vi "Slice Engine.vi"(7 "Table Stages":T3={"X Stage"={"Position"=0.0, "Is.Enabled?"=FALSE, "Is.Connected?"=FALSE, "Device SN"="45876425", "AccelerationMaximum"=20.0, "VelocityMaximum"=20.0, "Acceleration"=15.0, "Velocity"=18.0, "waitTimeout (ms)"=500000, "Model"=enum."None", "Is.Homed?"=FALSE, "MOVE"=FALSE}, "Y Stage"={"Position"=0.0, "Is.Enabled?"=FALSE, "Is.Connected?"=FALSE, "Device SN"="45995820", "AccelerationMaximum"=20.0, "VelocityMaximum"=20.0, "Acceleration"=15.0, "Velocity"=18.0, "waitTimeout (ms)"=5000000, "Model"=enum."None", "Is.Homed?"=FALSE, "MOVE"=FALSE}, "Z Stage"={"Position"=0.0, "Is.Enabled?"=FALSE, "Is.Connected?"=FALSE, "Device SN"="49103464", "AccelerationMaximum"=0.0, "VelocityMaximum"=0.0, "Acceleration"=0.0, "Velocity"=0.0, "waitTimeout (ms)"=0, "Model"=enum."None", "Is.Homed?"=FALSE, "MOVE"=FALSE}, "Attenuator"={"Position"=0.0, "Is.Enabled?"=FALSE, "Is.Connected?"=FALSE, "Device SN"="45876539", "AccelerationMaximum"=0.0, "VelocityMaximum"=0.0, "Acceleration"=0.0, "Velocity"=0.0, "waitTimeout (ms)"=0, "Model"=enum."None", "Is.Homed?"=FALSE, "MOVE"=FALSE}}, 8 "error in (no error)":errorcluster, 9 "Vibratome":T1={"Pre Cut Dwell [s]"=0.0, "Blade Frequency [RPM]"=0, "Slice Speed [mm/s]"=0.0, "Post Cut Dwell [s]"=0.0, "Ramp Time [s]"=0.0, "Start X [mm]"=0.0, "Start Y [mm]"=0.0, "Slice Length [mm]"=0.0, "Slice Axis"=enum."X Axis", "Controller VISA Ref"="COM4", "Blade Frequency [Hz]"=0, "Analog Out Channel"="GalvoCtrl/ao0,GalvoCtrl/ao1", "Pixel Clock Source"="/GalvoCtrl/PFI0", "Vib version"=enum."Vibratome1"}, 10 "Action":string="Init", 11 "Last Slice?":bool) -> (0 "error out":errorcluster)   [LabVIEW 2018]
uses:
  Controls/Translation Stage Parameters.ctl
  Hardware Mfg/Thorlabs Translation Stages/Controls/Translation Stage Cluster.ctl
  Controls/Translation Stage Types.ctl
  Controls/Vibratome Parameters.ctl
  type defines/vibratome.ctl
  Controls/Queue Manager Actions.ctl
  Controls/QueueNames.ctl
  Controls/Set Get Controls.ctl
  Hardware Mfg/Thorlabs Translation Stages/Controls/Motion Translation Module Control2.ctl
  Controls/FGV Actions.ctl
  Hardware Mfg/Thorlabs Translation Stages/Controls/Motion Translation Module Control.ctl
  Controls/vibratome3 control.ctl
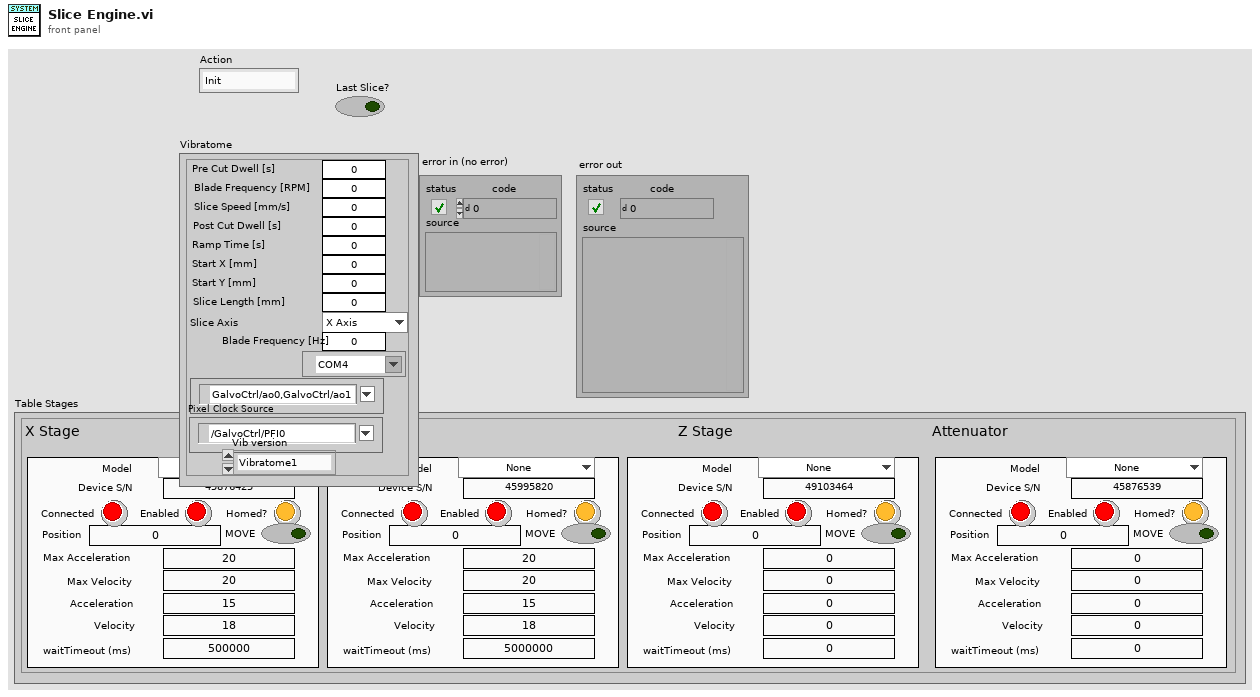
[diagram p1: front panel]
types:
  T1 = typedef "Vibratome Parameters.ctl" = cluster{"Pre Cut Dwell [s]":dbl, "Blade Frequency [RPM]":u16, "Slice Speed [mm/s]":dbl, "Post Cut Dwell [s]":dbl, "Ramp Time [s]":dbl, "Start X [mm]":dbl, "Start Y [mm]":dbl, "Slice Length [mm]":dbl, "Slice Axis":enum16{"X Axis", "Y Axis", "Z Axis"}, "Controller VISA Ref":refnum<visa-resource-name>, "Blade Frequency [Hz]":u16, "Analog Out Channel":tag, "Pixel Clock Source":tag, "Vib version":T2}
  T2 = typedef "vibratome.ctl" = enum16{"Vibratome1", "Vibratome3"}
  T3 = typedef "Translation Stage Parameters.ctl" = cluster{"X Stage":T4, "Y Stage":T4, "Z Stage":T4, "Attenuator":T4}
  T4 = typedef "Translation Stage Cluster.ctl" = cluster{"Position":dbl, "Is.Enabled?":bool, "Is.Connected?":bool, "Device SN":string, "AccelerationMaximum":dbl, "VelocityMaximum":dbl, "Acceleration":dbl, "Velocity":dbl, "waitTimeout (ms)":i32, "Model":T5, "Is.Homed?":bool, "MOVE":bool}
  T5 = typedef "Translation Stage Types.ctl" = enum16{"None", "Thorlabs LTS", "Thorlabs MLJ"}
  T6 = typedef "QueueNames.ctl" = enum16{"Main GUI", "Main Scan Processor", "Main Processing", "Main Saving", "Main Display", "Main Table Stage GUI", "Main Table Stage Proc.", "Scan Engine", "Vibratome GUI", "Vibratome Processor", "Slice Engine"}
  T7 = typedef "Queue Manager Actions.ctl" = enum16{"Init", "Enqueue", "Enqueue All", "Preview Queue", "Dequeue", "Get Status", "Flush Queue", "Flush All Queues", "Release All Queues", "Release Queue", "Enqueue at Opposite End"}
  T8 = typedef "Set Get Controls.ctl" = enum16{"Set", "Get"}
  T9 = typedef "Motion Translation Module Control.ctl" = enum16{"Init", "Home", "Status", "Velocity/Accel", "Position", "Jog", "Stop", "Uninit", "Enable", "Disable"}
  T10 = typedef "Motion Translation Module Control2.ctl" = enum16{"Init", "Home", "Status", "Velocity/Accel", "Position", "Jog", "Stop", "Uninit", "Enable", "Disable"}
  T11 = typedef "FGV Actions.ctl" = enum16{"Init", "Set", "Get", "Clear"}
  T12 = enum16{"Set Configuration", "Get Configuration", "Enable Motor", "Disable Motor", "Get Status", "Open Session", "Close Session", "Set Limits", "Get Limits"}
  T13 = cluster{"Source for Velocity":enum16{"Interface", "Voltage (AI)", "PWM (AI)", "Current Target (AI)", "Current Target w/ Preset (AI)"}, "Mode":enum16{"Continuous", "Stepper Motor", "Analog Position Ctrl", "Encoder"}, "Target Velocity [RPM]":i16}
  T14 = typedef "vibratome3 control.ctl" = enum16{"Init", "Configure channel", "Write waveform", "Start", "Stop", "Finish?", "Uninit"}
  T15 = typedef "Motion Translation Module Control.ctl" = enum16{"Uninit", "Measure power", "Move angle", "Gen angles", "Init cage", "Init PM"}
  T16 = typedef "MessagePacket.ctl" = cluster{"Message":string, "Parameter":variant}
  T17 = typedef "Translation Stage Quick Status.ctl" = cluster{"Is.Enabled?":bool, "Is.Connected?":bool, "Is.Homed?":bool}
  T18 = typedef "ScanType.ctl" = enum16{"Single Frame", "Continuous Frame", "ROI Line", "Vibratome", "Mosaic", "Mosaic + Slice"}
  T19 = enum16{"Left Button", "Center Button", "Right Button", "Window Close"}
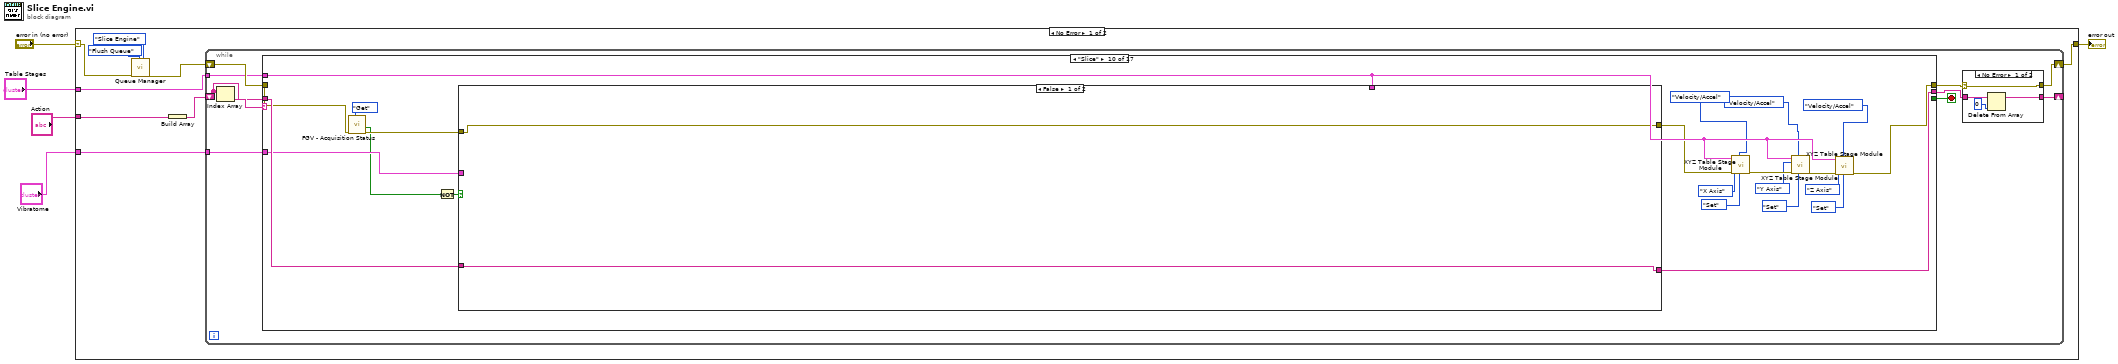
[diagram p0: block diagram]
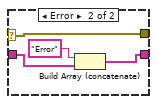
[diagram p2: hidden frame]
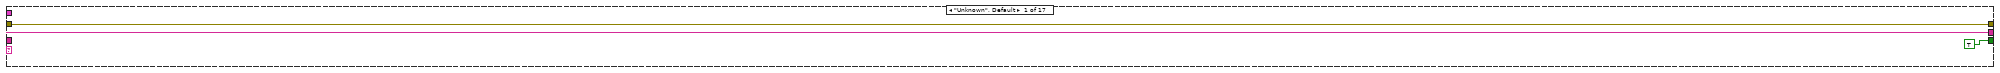
[diagram p3: hidden frame]
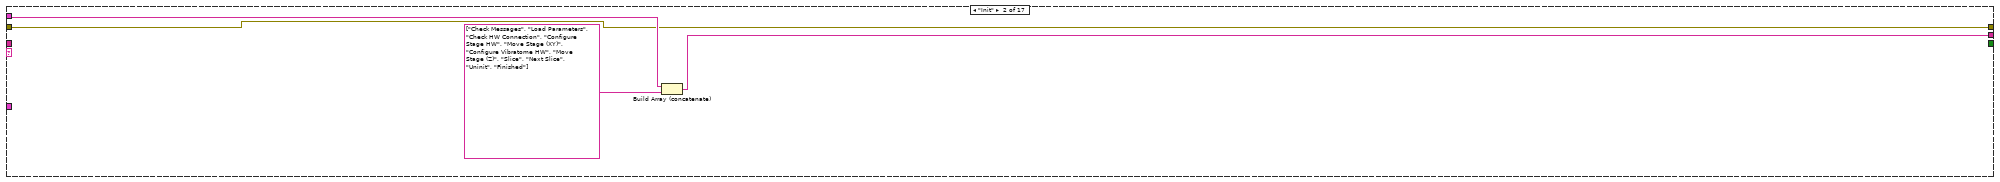
[diagram p4: hidden frame]
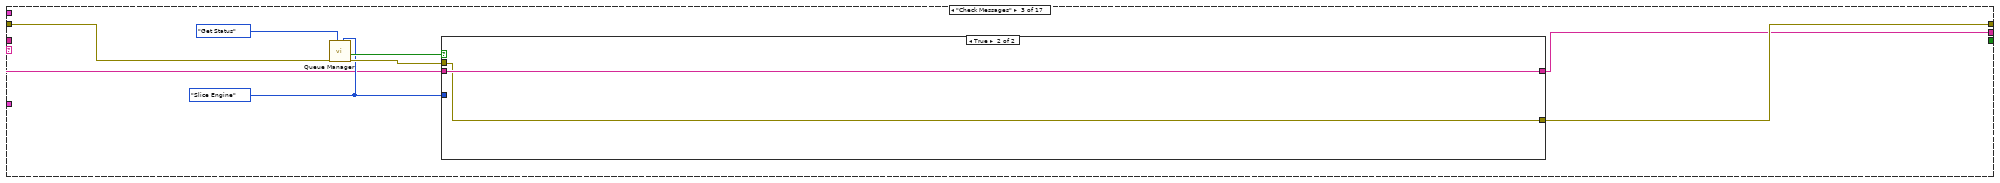
[diagram p5: hidden frame]
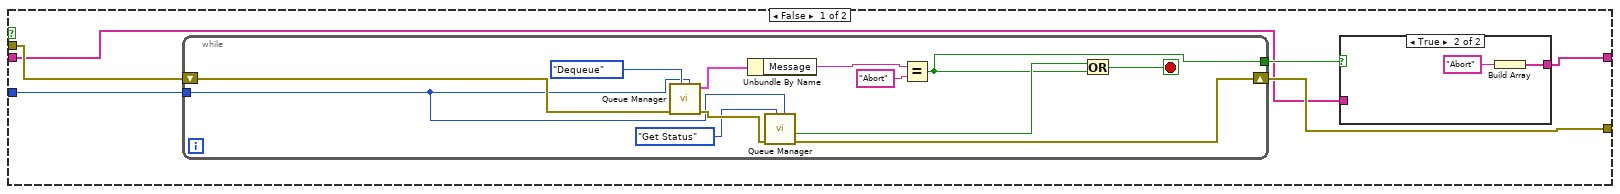
[diagram p6: hidden frame]
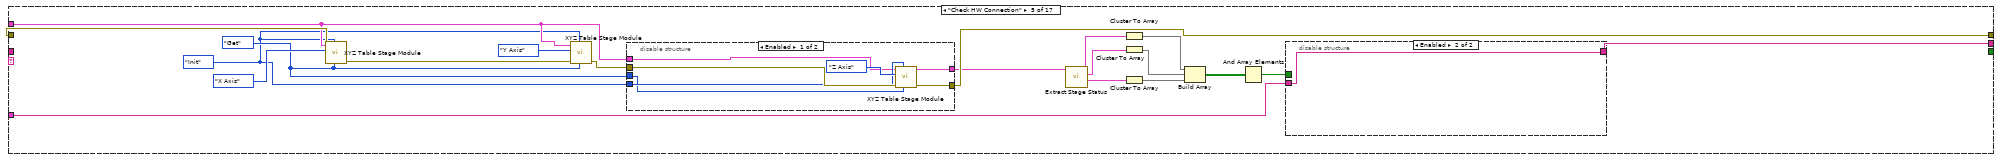
[diagram p9: hidden frame]
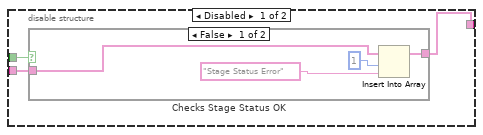
[diagram p10: hidden frame]
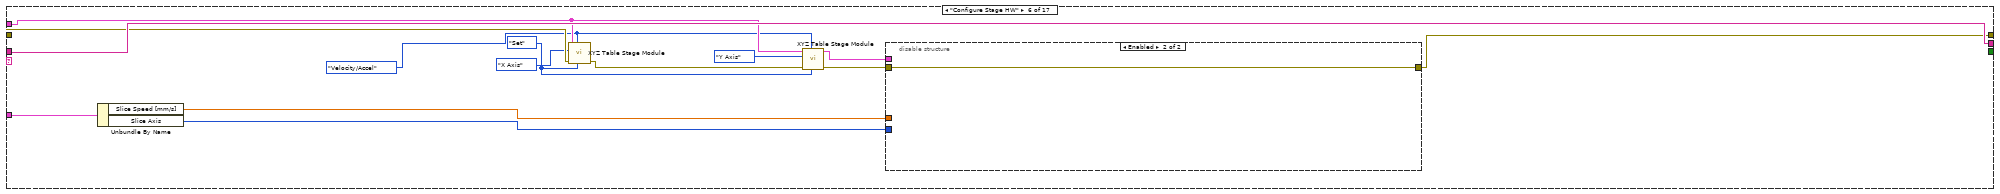
[diagram p13: hidden frame]
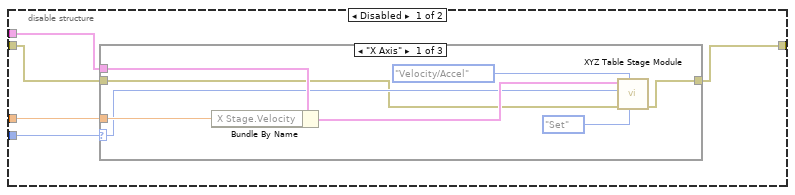
[diagram p14: hidden frame]
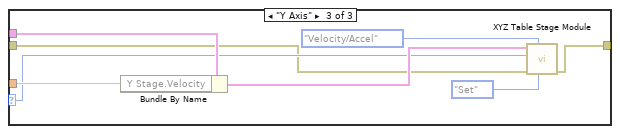
[diagram p16: hidden frame]
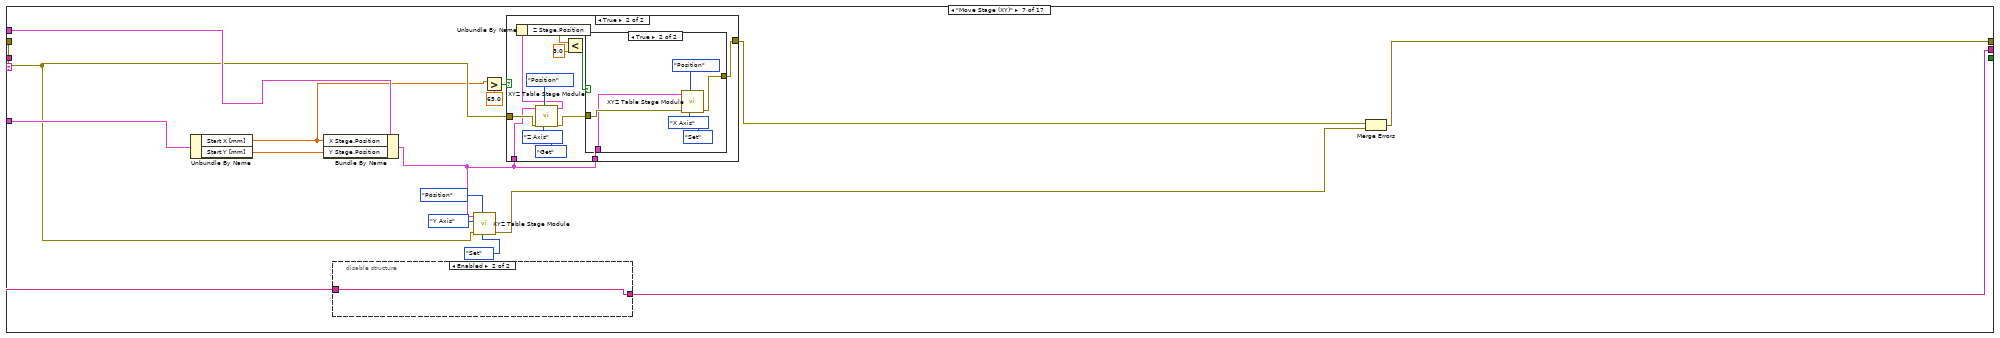
[diagram p17: hidden frame]
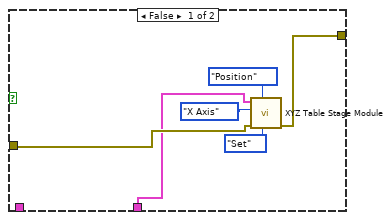
[diagram p18: hidden frame]
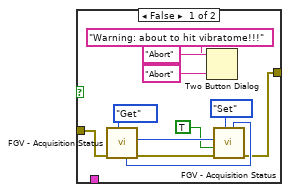
[diagram p19: hidden frame]
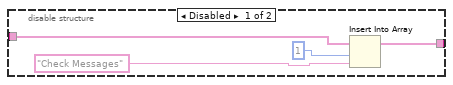
[diagram p20: hidden frame]
diagram:
  n1 = case shown="No Error" "error in (no error)" {
    selector: "error in (no error)" -> [w10 w540]
    tunnel: [w11 w540] -> w4
    tunnel: "Action" -> [w9 _]
    tunnel: "Table Stages" -> [w7 _]
    tunnel: "Vibratome" -> [w6 _]
    frame No Error {
      n2 = call "Queue Manager.vi"("Queue Name"=QueueNames."Slice Engine", "Action"=Queue_Manager_Actions."Flush Queue", "Error In"=w10) -> ("Error Out"=w8:errorcluster)  [unwired: 4 in, 4 out]
      n3 = Build Array(w9) -> (w12:string[])
      n4 = while {
        shift-right: [w19] -> _
        shift-left: w12 -> [w18]
        shift-right: [w21] -> w11
        shift-left: w8 -> [w24]
        tunnel: w7 -> [w17]
        tunnel: w6 -> [w16]
        stop <- w15 stop-if-true
        n5 = Index Array(array=w18) -> (element=w23:string)  [unwired: 1 in]
        n6 = case shown="\"Slice\"" w23 {
          tunnel: w24 -> [w34 w36 w47 w71 w92 w123 w151 w210 w214 w238 w333 w376 w394 w418 w422 w451 w538]
          tunnel: w18 -> [w35 w39 w41 w72 w76 w124 w163 w211 w213 w241 w336 w379 w391 w415 w420 w452 w539]
          tunnel: [w35 w38 w40 w72 w77 w124 w162 w211 w212 w240 w335 w378 w391 w416 w419 w452 w539] -> w20
          tunnel: [w34 w36 w42 w71 w91 w114 w161 w204 w214 w239 w334 w376 w392 w418 w423 w450 w537] -> w22
          tunnel: w17 -> [_ _ _ _ w74 w113 w160 _ _ w236 w331 _ w390 _ _ w449 _]
          tunnel: w16 -> [_ _ _ _ _ w112 w159 w206 _ w237 w332 _ w389 _ _ _ _]
          tunnel: [TRUE _ _ _ _ _ _ _ _ _ _ _ _ _ _ _ TRUE] -> w15
          frame "Unknown", Default {
          }
          frame "Init" {
            n7 = Build Array (concatenate)(w39, string[] ["Check Messages", "Load Parameters", "Check HW Connection", "Configure Stage HW", "Move Stage (XY)", "Configure Vibratome HW", "Move Stage (Z)", "Slice", "Next Slice", "Uninit", "Finished"]) -> (w38:string[])
          }
          frame "Check Messages" {
            w43 = QueueNames."Slice Engine" ("Queue Name")
            n8 = call "Queue Manager.vi"("Queue Name"=w43, "Action"=Queue_Manager_Actions."Get Status", "Error In"=w47) -> ("Error Out"=w44:errorcluster, "Empty?"=w45:bool)  [unwired: 4 in, 3 out]
            n9 = case shown="True" w45 {
              tunnel: w44 -> [w53 w69]
              tunnel: w43 -> [w52 _]
              tunnel: [w51 w69] -> w42
              tunnel: w41 -> [w49 w70]
              tunnel: [w48 w70] -> w40
              frame False {
                n10 = while {
                  tunnel: w52 -> [w64]
                  shift-right: [w65] -> w51
                  shift-left: w53 -> [w68]
                  tunnel: [w57] -> w50
                  stop <- w58 stop-if-true
                  n11 = call "Queue Manager.vi"("Queue Name"=w64, "Action"=Queue_Manager_Actions."Dequeue", "Error In"=w68) -> ("Error Out"=w66:errorcluster, "Message Packet [Out]"=w62:T16)  [unwired: 4 in, 3 out]
                  n12 = Unbundle By Name(w62) -> ("Message"=w61:string)
                  n13 = call "Queue Manager.vi"("Queue Name"=w64, "Action"=Queue_Manager_Actions."Get Status", "Error In"=w66) -> ("Error Out"=w65:errorcluster, "Empty?"=w59:bool)  [unwired: 4 in, 3 out]
                  n14 = Equal?(x=w61, y="Abort") -> (x = y?=w57:bool)
                  n15 = Or(x=w59, y=w57) -> (x .or. y?=w58:bool)
                }
                n16 = case shown="True" w50 {
                  tunnel: w49 -> [w54 _]
                  tunnel: [w54 w55] -> w48
                  frame False {
                  }
                  frame True {
                    n17 = Build Array("Abort") -> (w55:string[])
                  }
                }
              }
              frame True {
              }
            }
          }
          frame "Load Parameters" {
          }
          frame "Check HW Connection" {
            w73 = Motion_Translation_Module_Control2."Init" ("Action")
            w86 = Set_Get_Controls."Get" ("Set/Get")
            n18 = call "XYZ Table Stage Module.vi"("Set/Get"=w86, "Action"=w73, "Error In"=w92, "Axis"=enum16{"X Axis", "Y Axis", "Z Axis"}."X Axis", "Table Stages"=w74) -> ("Error Out"=w90:errorcluster)  [unwired: 5 in, 1 out]
            n19 = call "XYZ Table Stage Module.vi"("Set/Get"=w86, "Action"=w73, "Error In"=w90, "Axis"=enum16{"X Axis", "Y Axis", "Z Axis"}."Y Axis", "Table Stages"=w74) -> ("Error Out"=w89:errorcluster)  [unwired: 5 in, 1 out]
            n20 = disable-structure shown="Enabled" {
              disable-tunnel: [w108 w110] -> w91
              disable-tunnel: w89 -> [w107 w110]
              disable-tunnel: w73 -> [w105 _]
              disable-tunnel: w86 -> [w104 _]
              disable-tunnel: w74 -> [w103 w109]
              disable-tunnel: [w102 w109] -> w85
              frame Enabled {
                n21 = call "XYZ Table Stage Module.vi"("Set/Get"=w104, "Action"=w105, "Error In"=w107, "Axis"=enum16{"X Axis", "Y Axis", "Z Axis"}."Z Axis", "Table Stages"=w103) -> ("Error Out"=w108:errorcluster, "Table Stages [out]"=w102:T3)  [unwired: 5 in]
              }
              frame Disabled {
              }
            }
            n22 = call "Extract Stage Status.vi"("Table Stages"=w85) -> ("Z Stage"=w82:T17, "Y Stage"=w83:T17, "X Stage"=w84:T17)  [unwired: 8 in]
            n23 = Cluster To Array(cluster=w84) -> (array=w81:bool[])
            n24 = Cluster To Array(cluster=w83) -> (array=w80:bool[])
            n25 = Cluster To Array(cluster=w82) -> (array=w79:bool[])
            n26 = Build Array(w81, w80, w79) -> (w78:bool[][])
            n27 = And Array Elements(Boolean array=w78) -> (logical AND=w75:bool)
            n28 = disable-structure shown="Enabled" {
              disable-tunnel: [w95 w101] -> w77
              disable-tunnel: w76 -> [w94 w101]
              disable-tunnel: w75 -> [w93 _]
              frame Disabled {
                n29 = case "Checks Stage Status OK" shown="False" w93 {
                  tunnel: [w99 w100] -> w95
                  tunnel: w94 -> [w98 w100]
                  frame False {
                    n30 = Insert Into Array(array=w98, index=1, new element="Stage Status Error" ("new element/subarray")) -> (w99:string[])
                  }
                  frame True {
                  }
                }
              }
              frame Enabled {
              }
            }
          }
          frame "Configure Stage HW" {
            w111 = Motion_Translation_Module_Control2."Velocity/Accel" ("Action")
            w119 = Set_Get_Controls."Set" ("Set/Get")
            n31 = Unbundle By Name(w112) -> ("Slice Speed [mm/s]"=w117:dbl, "Slice Axis"=w118:enum16{"X Axis", "Y Axis", "Z Axis"})
            n32 = call "XYZ Table Stage Module.vi"("Set/Get"=w119, "Action"=w111, "Error In"=w123, "Axis"=enum16{"X Axis", "Y Axis", "Z Axis"}."X Axis", "Table Stages"=w113) -> ("Error Out"=w122:errorcluster)  [unwired: 5 in, 1 out]
            n33 = call "XYZ Table Stage Module.vi"("Set/Get"=w119, "Action"=w111, "Error In"=w122, "Axis"=enum16{"X Axis", "Y Axis", "Z Axis"}."Y Axis", "Table Stages"=w113) -> ("Error Out"=w115:errorcluster, "Table Stages [out]"=w116:T3)  [unwired: 5 in]
            n34 = disable-structure shown="Enabled" {
              disable-tunnel: w118 -> [w129 _]
              disable-tunnel: w117 -> [w128 _]
              disable-tunnel: w116 -> [w127 _]
              disable-tunnel: w115 -> [w126 w147]
              disable-tunnel: [w125 w147] -> w114
              frame Disabled {
                n35 = case shown="\"X Axis\"" w129 {
                  selector: w129 -> [w134 _ w143]
                  tunnel: w128 -> [w137 _ w146]
                  tunnel: w127 -> [w136 _ w145]
                  tunnel: w126 -> [w133 w138 w142]
                  tunnel: [w132 w138 w141] -> w125
                  frame "X Axis" {
                    n36 = Bundle By Name(cluster=w136, "X Stage.Velocity"=w137) -> (w135:T3)
                    n37 = call "XYZ Table Stage Module.vi"("Set/Get"=Set_Get_Controls."Set", "Action"=Motion_Translation_Module_Control."Velocity/Accel", "Error In"=w133, "Axis"=w134, "Table Stages"=w135) -> ("Error Out"=w132:errorcluster)  [unwired: 5 in, 1 out]
                  }
                  frame "Z Axis" {
                  }
                  frame "Y Axis" {
                    n38 = Bundle By Name(cluster=w145, "Y Stage.Velocity"=w146) -> (w144:T3)
                    n39 = call "XYZ Table Stage Module.vi"("Set/Get"=Set_Get_Controls."Set", "Action"=Motion_Translation_Module_Control."Velocity/Accel", "Error In"=w142, "Axis"=w143, "Table Stages"=w144) -> ("Error Out"=w141:errorcluster)  [unwired: 5 in, 1 out]
                  }
                }
              }
              frame Enabled {
              }
            }
          }
          frame "Move Stage (XY)" {
            n40 = Unbundle By Name(w159) -> ("Start X [mm]"=w150:dbl, "Start Y [mm]"=w157:dbl)
            n41 = Bundle By Name(cluster=w160, "X Stage.Position"=w150, "Y Stage.Position"=w157) -> (w149:T3)
            n42 = disable-structure shown="Enabled" {
              disable-tunnel: w163 -> [w202 w203]
              disable-tunnel: [w201 w203] -> w162
              frame Disabled {
                n43 = Insert Into Array(array=w202, index=1, new element="Check Messages" ("new element/subarray")) -> (w201:string[])
              }
              frame Enabled {
              }
            }
            n44 = call "XYZ Table Stage Module.vi"("Set/Get"=Set_Get_Controls."Set", "Action"=Motion_Translation_Module_Control2."Position", "Error In"=w151, "Axis"=enum16{"X Axis", "Y Axis", "Z Axis"}."Y Axis", "Table Stages"=w149) -> ("Error Out"=w158:errorcluster)  [unwired: 5 in, 1 out]
            n45 = Greater?(x=w150, y=65.0) -> (0:w153:bool)
            n46 = case shown="True" w153 {
              tunnel: w151 -> [w165 w173]
              tunnel: w149 -> [_ w172]
              tunnel: [w166 w179] -> w148
              tunnel: w149 -> [w164 w178]
              frame False {
                n47 = call "XYZ Table Stage Module.vi"("Set/Get"=Set_Get_Controls."Set", "Action"=Motion_Translation_Module_Control2."Position", "Error In"=w165, "Axis"=enum16{"X Axis", "Y Axis", "Z Axis"}."X Axis", "Table Stages"=w164) -> ("Error Out"=w166:errorcluster)  [unwired: 5 in, 1 out]
              }
              frame True {
                n48 = call "XYZ Table Stage Module.vi"("Set/Get"=Set_Get_Controls."Get", "Action"=Motion_Translation_Module_Control2."Position", "Error In"=w173, "Axis"=enum16{"X Axis", "Y Axis", "Z Axis"}."Z Axis", "Table Stages"=w172) -> ("Error Out"=w171:errorcluster, "Table Stages [out]"=w170:T3)  [unwired: 5 in]
                n49 = Unbundle By Name(w170) -> ("Z Stage.Position"=w177:dbl)
                n50 = Less?(x=w177, y=3.0) -> (x < y?=w180:bool)
                n51 = case shown="True" w180 {
                  tunnel: w171 -> [w183 w194]
                  tunnel: [w182 w195] -> w179
                  tunnel: w178 -> [_ w193]
                  frame False {
                    n52 = call "FGV - Acquisition Status.vi"("Actions"=FGV_Actions."Get", "Error In"=w183) -> ("Error Out"=w186:errorcluster, "Scan Type [Out]"=w187:T18, "mem loc out"=w184:i32)  [unwired: 6 in, 1 out]
                    n53 = Two Button Dialog(message="Warning: about to hit vibratome!!!" ("T button name (\"OK\")"), 1:"Abort" ("F button name (\"Cancel\")"), 2:"Abort" ("T button name (\"OK\")")) -> ()  [unwired: 1 out]
                    n54 = call "FGV - Acquisition Status.vi"("mem loc"=w184, "Actions"=FGV_Actions."Set", "Error In"=w186, "Quit status"=TRUE, "Scan Type [In]"=w187) -> ("Error Out"=w182:errorcluster)  [unwired: 3 in, 3 out]
                  }
                  frame True {
                    n55 = call "XYZ Table Stage Module.vi"("Set/Get"=Set_Get_Controls."Set", "Action"=Motion_Translation_Module_Control2."Position", "Error In"=w194, "Axis"=enum16{"X Axis", "Y Axis", "Z Axis"}."X Axis", "Table Stages"=w193) -> ("Error Out"=w195:errorcluster)  [unwired: 5 in, 1 out]
                  }
                }
              }
            }
            n56 = Merge Errors(w148, w158) -> (w161:errorcluster)
          }
          frame "Configure Vibratome HW" {
            n57 = Unbundle By Name(w206) -> ("Controller VISA Ref"=w205:refnum<visa-resource-name>)
            n58 = call "MCDC3006 Module.vi"("Actions"=T12."Open Session", "Error In"=w210, "VISA resource name"=w205) -> ("Error Out"=w207:errorcluster)  [unwired: 4 in, 4 out]
            n59 = call "MCDC3006 Module.vi"("Actions"=T12."Enable Motor", "Error In"=w207, "VISA resource name"=w205) -> ("Error Out"=w204:errorcluster)  [unwired: 4 in, 4 out]
          }
          frame "Move Stage (Z)" {
            n60 = disable-structure shown="Disabled" {
              disable-tunnel: w213 -> [w218 w219]
              disable-tunnel: [w217 w219] -> w212
              frame Disabled {
                n61 = Insert Into Array(array=w218, index=1, new element="Check Messages" ("new element/subarray")) -> (w217:string[])
              }
              frame Enabled {
              }
            }
          }
          frame "Slice" {
            n62 = call "FGV - Acquisition Status.vi"("Actions"=FGV_Actions."Get", "Error In"=w238) -> ("Error Out"=w222:errorcluster, "Quit status out"=w220:bool)  [unwired: 6 in, 2 out]
            n63 = Not(x=w220) -> (.not. x?=w221:bool)
            n64 = case shown="False" w221 {
              tunnel: w241 -> [w242 w263]
              tunnel: [w242 w262] -> w240
              tunnel: w237 -> [_ w261]
              tunnel: w236 -> [_ w260]
              tunnel: [w243 w245] -> w227
              tunnel: w222 -> [w243 w244]
              frame False {
              }
              frame True {
                n65 = Unbundle By Name(w261) -> ("Controller VISA Ref"=w246:refnum<visa-resource-name>, "Blade Frequency [RPM]"=w254:u16, "Slice Axis"=w259:enum16{"X Axis", "Y Axis", "Z Axis"}, "Slice Length [mm]"=w258:dbl, "Post Cut Dwell [s]"=w252:dbl, "Pre Cut Dwell [s]"=w251:dbl, "Slice Speed [mm/s]"=w250:dbl, "Start X [mm]"=w247:dbl)
                n66 = disable-structure shown="Enabled" {
                  disable-tunnel: w263 -> [w305 w306]
                  disable-tunnel: [w304 w306] -> w262
                  frame Disabled {
                    n67 = Insert Into Array(array=w305, index=1, new element="Check Messages" ("new element/subarray")) -> (w304:string[])
                  }
                  frame Enabled {
                  }
                }
                n68 = Bundle By Name(cluster=T13 {"Source for Velocity"=enum."Interface", "Mode"=enum."Continuous", "Target Velocity [RPM]"=0} ("Configuration [In]"), "Target Velocity [RPM]"=w254) -> (w253:T13)
                n69 = call "MCDC3006 Module.vi"("Actions"=T12."Enable Motor", "Error In"=w244, "VISA resource name"=w246) -> ("Error Out"=w248:errorcluster)  [unwired: 4 in, 4 out]
                n70 = call "MCDC3006 Module.vi"("Actions"=T12."Set Configuration", "Error In"=w248, "Configuration [In]"=w253, "VISA resource name"=w246) -> ("Error Out"=w257:errorcluster)  [unwired: 3 in, 4 out]
                n71 = case shown="\"X Axis\"" w259 {
                  tunnel: w257 -> [w284 w285 w301]
                  tunnel: [w275 w285 w288] -> w245
                  tunnel: w258 -> [w278 _ w295]
                  tunnel: w252 -> [w273 _ w291]
                  tunnel: w251 -> [w281 _ _]
                  tunnel: w250 -> [_ _ _]
                  tunnel: w247 -> [w268 _ _]
                  tunnel: w260 -> [w265 _ _]
                  frame "X Axis" {
                    n72 = expression code="x*1000"(w281) -> (w280:dbl)
                    n73 = To Unsigned Long Integer(number=w280) -> (unsigned 32bit integer=w279:u32)
                    n74 = call "Inline Wait.vi"("Error In"=w284, "milliseconds to wait"=w279) -> ("Error Out"=w270:errorcluster)  [unwired: 9 in]
                    n75 = Multiply(x=w273, y=1000.0) -> (x*y=w276:dbl)
                    n76 = Subtract(x=w268, y=w278) -> (x-y=w283:dbl)
                    n77 = To Unsigned Long Integer(number=w276) -> (unsigned 32bit integer=w282:u32)
                    n78 = Bundle By Name(cluster=w265, "X Stage.Position"=w283) -> (w267:T3)
                    n79 = call "XYZ Table Stage Module.vi"("Set/Get"=Set_Get_Controls."Set", "Action"=Motion_Translation_Module_Control2."Position", "Error In"=w270, "Axis"=enum16{"X Axis", "Y Axis", "Z Axis"}."X Axis", "Table Stages"=w267) -> ("Error Out"=w269:errorcluster)  [unwired: 5 in, 1 out]
                    n80 = call "Inline Wait.vi"("Error In"=w269, "milliseconds to wait"=w282) -> ("Error Out"=w266:errorcluster)  [unwired: 9 in]
                    n81 = call "MCDC3006 Module.vi"("Actions"=T12."Disable Motor", "Error In"=w266) -> ("Error Out"=w275:errorcluster)  [unwired: 5 in, 4 out]
                  }
                  frame "Z Axis" {
                  }
                  frame "Y Axis" {
                    (unwired) Motion_Translation_Module_Control."Init cage" ("Action")
                    n82 = expression code="x*1000"(w291) -> (w290:dbl)
                    n83 = call "Thorlabs LTS - Y Stage Module.vi"("Set/Get"=Set_Get_Controls."Get", "Error In"=w301) -> ("Error Out"=w300:errorcluster, "Cluster Out"=w286:T4)  [unwired: 8 in]
                    n84 = Unbundle By Name(w286) -> ("Position"=w296:dbl)
                    n85 = To Unsigned Long Integer(number=w290) -> (unsigned 32bit integer=w289:u32)
                    n86 = Add(x=w296, y=w295) -> (x+y=w294:dbl)
                    n87 = Bundle By Name(cluster=w286, "Position"=w294) -> (w293:T4)
                    n88 = call "Thorlabs LTS - Y Stage Module.vi"("Set/Get"=Set_Get_Controls."Set", "Error In"=w300, "Cluster In"=w293) -> ("Error Out"=w298:errorcluster)  [unwired: 7 in, 1 out]
                    n89 = call "Inline Wait.vi"("Error In"=w298, "milliseconds to wait"=w289) -> ("Error Out"=w292:errorcluster)  [unwired: 9 in]
                    n90 = call "Thorlabs LTS - Y Stage Module.vi"("Set/Get"=Set_Get_Controls."Set", "Error In"=w292, "Cluster In"=w286) -> ("Error Out"=w288:errorcluster)  [unwired: 7 in, 1 out]
                  }
                }
              }
            }
            n91 = call "XYZ Table Stage Module.vi"("Set/Get"=Set_Get_Controls."Set", "Action"=Motion_Translation_Module_Control2."Velocity/Accel", "Error In"=w227, "Axis"=enum16{"X Axis", "Y Axis", "Z Axis"}."X Axis", "Table Stages"=w236) -> ("Error Out"=w235:errorcluster)  [unwired: 5 in, 1 out]
            n92 = call "XYZ Table Stage Module.vi"("Set/Get"=Set_Get_Controls."Set", "Action"=Motion_Translation_Module_Control2."Velocity/Accel", "Error In"=w235, "Axis"=enum16{"X Axis", "Y Axis", "Z Axis"}."Y Axis", "Table Stages"=w236) -> ("Error Out"=w230:errorcluster)  [unwired: 5 in, 1 out]
            n93 = call "XYZ Table Stage Module.vi"("Set/Get"=Set_Get_Controls."Set", "Action"=Motion_Translation_Module_Control2."Velocity/Accel", "Error In"=w230, "Axis"=enum16{"X Axis", "Y Axis", "Z Axis"}."Z Axis", "Table Stages"=w236) -> ("Error Out"=w239:errorcluster)  [unwired: 5 in, 1 out]
          }
          frame "Slice3" {
            n94 = disable-structure shown="Enabled" {
              disable-tunnel: w336 -> [w374 w375]
              disable-tunnel: [w373 w375] -> w335
              frame Disabled {
                n95 = Insert Into Array(array=w374, index=1, new element="Check Messages" ("new element/subarray")) -> (w373:string[])
              }
              frame Enabled {
              }
            }
            n96 = Unbundle By Name(w332) -> ("Slice Axis"=w329:enum16{"X Axis", "Y Axis", "Z Axis"}, "Slice Length [mm]"=w328:dbl, "Ramp Time [s]"=w308:dbl, "Slice Speed [mm/s]"=w327:dbl, "Start X [mm]"=w326:dbl, "Start Y [mm]"=w307:dbl)  [unwired: 1 out]
            n97 = flat-sequence {
              tunnel: w333 -> [w345]
              tunnel: [w337] -> w330
              tunnel: [w349] -> w314
              tunnel: w330 -> [w349]
              tunnel: w308 -> [w346]
              frame #0 {
                n98 = call "vibratome3 module.vi"("Action"=vibratome3_control."Init", "error in"=w345) -> ("error out"=w340:errorcluster)  [unwired: 9 in]
                n99 = call "vibratome3 module.vi"("Action"=vibratome3_control."Configure channel", "error in"=w340) -> ("error out"=w339:errorcluster)  [unwired: 9 in]
                n100 = call "vibratome3 module.vi"("Action"=vibratome3_control."Write waveform", "error in"=w339) -> ("error out"=w338:errorcluster)  [unwired: 9 in]
                n101 = call "vibratome3 module.vi"("Action"=vibratome3_control."Start", "error in"=w338) -> ("error out"=w337:errorcluster)  [unwired: 9 in]
              }
              frame #1 {
                n102 = Multiply(x=w346, y=1000.0) -> (x*y=w348:dbl)
                n103 = Wait (ms)(milliseconds to wait=w348) -> ()  [unwired: 1 out]
              }
            }
            n104 = case shown="\"Y Axis\"" w329 {
              tunnel: w314 -> [w350 w361 w370]
              tunnel: [w351 w362 w370] -> w310
              tunnel: w328 -> [w358 w368 _]
              tunnel: w327 -> [_ _ _]
              tunnel: w326 -> [w355 _ _]
              tunnel: w331 -> [w353 w364 _]
              tunnel: w307 -> [_ w360 _]
              frame "X Axis", Default {
                n105 = Subtract(x=w355, y=w358) -> (x-y=w359:dbl)
                n106 = Bundle By Name(cluster=w353, "X Stage.Position"=w359) -> (w354:T3)
                n107 = call "XYZ Table Stage Module.vi"("Set/Get"=Set_Get_Controls."Set", "Action"=Motion_Translation_Module_Control2."Position", "Error In"=w350, "Axis"=enum16{"X Axis", "Y Axis", "Z Axis"}."X Axis", "Table Stages"=w354) -> ("Error Out"=w351:errorcluster)  [unwired: 5 in, 1 out]
              }
              frame "Y Axis" {
                n108 = Subtract(x=w360, y=w368) -> (x-y=w369:dbl)
                n109 = Bundle By Name(cluster=w364, "Y Stage.Position"=w369) -> (w365:T3)
                n110 = call "XYZ Table Stage Module.vi"("Set/Get"=Set_Get_Controls."Set", "Action"=Motion_Translation_Module_Control2."Position", "Error In"=w361, "Axis"=enum16{"X Axis", "Y Axis", "Z Axis"}."Y Axis", "Table Stages"=w365) -> ("Error Out"=w362:errorcluster)  [unwired: 5 in, 1 out]
              }
              frame "Z Axis" {
              }
            }
            n111 = call "vibratome3 module.vi"("Action"=vibratome3_control."Finish?", "error in"=w310) -> ("error out"=w311:errorcluster)  [unwired: 9 in]
            n112 = call "vibratome3 module.vi"("Action"=vibratome3_control."Uninit", "error in"=w311) -> ("error out"=w309:errorcluster)  [unwired: 9 in]
            n113 = call "XYZ Table Stage Module.vi"("Set/Get"=Set_Get_Controls."Set", "Action"=Motion_Translation_Module_Control2."Velocity/Accel", "Error In"=w309, "Axis"=enum16{"X Axis", "Y Axis", "Z Axis"}."X Axis", "Table Stages"=w331) -> ("Error Out"=w325:errorcluster)  [unwired: 5 in, 1 out]
            n114 = call "XYZ Table Stage Module.vi"("Set/Get"=Set_Get_Controls."Set", "Action"=Motion_Translation_Module_Control2."Velocity/Accel", "Error In"=w325, "Axis"=enum16{"X Axis", "Y Axis", "Z Axis"}."Y Axis", "Table Stages"=w331) -> ("Error Out"=w320:errorcluster)  [unwired: 5 in, 1 out]
            n115 = call "XYZ Table Stage Module.vi"("Set/Get"=Set_Get_Controls."Set", "Action"=Motion_Translation_Module_Control2."Velocity/Accel", "Error In"=w320, "Axis"=enum16{"X Axis", "Y Axis", "Z Axis"}."Z Axis", "Table Stages"=w331) -> ("Error Out"=w334:errorcluster)  [unwired: 5 in, 1 out]
          }
          frame "Next Slice" {
            n116 = case shown="True" "Last Slice?" {
              tunnel: w379 -> [w383 w385]
              tunnel: [w382 w384] -> w378
              frame False {
                n117 = Insert Into Array(array=w383, index=1, new element=string[] ["Move Stage (Z)", "Slice", "Next Slice"]) -> (w382:string[])
              }
              frame True {
                n118 = Insert Into Array(array=w385, index=1, new element=string[] ["Configure Stage HW", "", ""]) -> (w384:string[])
              }
            }
          }
          frame "Set Slice Speed" {
            n119 = Unbundle By Name(w389) -> ("Slice Axis"=w388:enum16{"X Axis", "Y Axis", "Z Axis"}, "Slice Speed [mm/s]"=w393:dbl)
            n120 = case shown="\"Y Axis\"" w388 {
              tunnel: w394 -> [w400 w410]
              tunnel: w393 -> [w399 w411]
              tunnel: [w398 w407] -> w392
              tunnel: w390 -> [w397 w406]
              frame "X Axis", Default {
                n121 = Bundle By Name(cluster=w397, "X Stage.Velocity"=w399, "X Stage.Acceleration"=50.0 ("Acceleration")) -> (w396:T3)
                n122 = call "XYZ Table Stage Module.vi"("Set/Get"=Set_Get_Controls."Set", "Action"=Motion_Translation_Module_Control2."Velocity/Accel", "Error In"=w400, "Axis"=enum16{"X Axis", "Y Axis", "Z Axis"}."X Axis", "Table Stages"=w396) -> ("Error Out"=w398:errorcluster)  [unwired: 5 in, 1 out]
              }
              frame "Y Axis" {
                n123 = Bundle By Name(cluster=w406, "Y Stage.Velocity"=w411, "Y Stage.Acceleration"=50.0 ("Acceleration")) -> (w405:T3)
                n124 = call "XYZ Table Stage Module.vi"("Set/Get"=Set_Get_Controls."Set", "Action"=Motion_Translation_Module_Control2."Velocity/Accel", "Error In"=w410, "Axis"=enum16{"X Axis", "Y Axis", "Z Axis"}."Y Axis", "Table Stages"=w405) -> ("Error Out"=w407:errorcluster)  [unwired: 5 in, 1 out]
              }
            }
          }
          frame "Abort" {
            n125 = Insert Into Array(array=w415, index=1, new element #1="Uninit", new element #2="Finished") -> (w416:string[])
          }
          frame "Error" {
            n126 = Unbundle(w422) -> ("code"=w432:i32, "source"=w431:string)  [unwired: 1 out]
            n127 = control-ref of="This VI"() -> (w433:refnum<vi>)
            n128 = property class="VI"(reference=w433) -> ("Name"=w436:string, "Callers"=w438:string[])  [unwired: 1 in, 2 out]
            n129 = Array To Spreadsheet String(delimiter (Tab)=">", array=w438, 3:"%s" ("format string")) -> (spreadsheet string=w437:string)
            n130 = Format Into String(format string="VI Name: %s\nCallers: %s\nError Code: %d\nError Message: %s", initial string="The following error occurred:\n" ("message"), w436, w437, w432, w431) -> (resulting string=w430:string, error out=w424:errorcluster)  [unwired: 1 in]
            n131 = call <vilib>:"Clear Errors.vi"("error in (no error)"=w424) -> ()  [unwired: 5 in, 2 out]
            n132 = call <vilib>:"Three Button Dialog.vi"("Allow user to close window? (TRUE)"=FALSE, "Window Title (\"\")"="Error" ("Window Title (\"\")"), "Right Button Text (\"Cancel\")"="Abort" ("Right Button Text (\"Cancel\")"), "Center Button Text (\"No\")"="Retry" ("Center Button Text (\"No\")"), "Left Button Text (\"Yes\")"="Continue" ("Left Button Text (\"Yes\")"), "message"=w430) -> ("Which Button?"=w421:T19)  [unwired: 5 in]
            n133 = case shown="\"Right Button\"" w421 {
              tunnel: w420 -> [w443 w447 w448]
              tunnel: [w442 w446 w448] -> w419
              frame "Left Button", Default {
                # "Continue"
                n134 = Delete From Array(array=w443, index=0) -> (array with subset deleted=w442:string[])  [unwired: 1 in, 1 out]
              }
              frame "Right Button" {
                # "Abort"
                n135 = Insert Into Array(array=w447, index=1, new element="Abort") -> (w446:string[])
              }
              frame "Center Button" {
                # "Retry"
              }
            }
            n136 = call <vilib>:"Clear Errors.vi"("error in (no error)"=w422) -> ("error out"=w423:errorcluster)  [unwired: 5 in, 1 out]
          }
          frame "Uninit" {
            n137 = disable-structure shown="Enabled" {
              disable-tunnel: w451 -> [w456 w534]
              disable-tunnel: [w455 w527] -> w450
              disable-tunnel: w449 -> [w453 _]
              frame Enabled {
                n138 = for {
                  N: 4 -> [_]
                  tunnel: [w462] -> w457 mode=indexing
                  tunnel: Motion_Translation_Module_Control."Uninit" ("Action") -> [w461]
                  tunnel: w456 -> [w460]
                  tunnel: w453 -> [w459]
                  i -> [w463]
                  n139 = case shown="3" w463 {
                    tunnel: [w467 w485 w503 w519] -> w462
                    tunnel: w460 -> [w466 w484 w502 w518]
                    tunnel: w461 -> [w465 w483 w501 _]
                    tunnel: w459 -> [w464 w482 w500 _]
                    frame 0, Default {
                      # "X Stage"
                      n140 = disable-structure shown="Enabled" {
                        disable-tunnel: [w473 _] -> w467
                        disable-tunnel: w466 -> [w472 _]
                        disable-tunnel: w465 -> [w471 _]
                        disable-tunnel: w464 -> [w468 _]
                        frame Disabled {
                          n141 = Unbundle By Name(w468) -> ("X Stage.Model"=w470:T5, "X Stage.Device SN"=w469:string)
                          n142 = case shown="\"Thorlabs LTS\"" w470 {
                            tunnel: [w474 w481] -> w473
                            tunnel: w472 -> [w474 w480]
                            tunnel: w471 -> [_ w479]
                            tunnel: w469 -> [_ w477]
                            frame "None", Default {
                            }
                            frame "Thorlabs LTS" {
                              n143 = Bundle By Name(cluster=T4 {"Position"=0.0, "Is.Enabled?"=TRUE, "Is.Connected?"=FALSE, "Device SN"="45876539", "AccelerationMaximum"=0.0, "VelocityMaximum"=0.0, "Acceleration"=0.0, "Velocity"=0.0, "waitTimeout (ms)"=0, "Model"=enum."Thorlabs LTS", "Is.Homed?"=FALSE, "MOVE"=FALSE} ("Cluster In"), "Device SN"=w477) -> (w476:T4)
                              n144 = call "Thorlabs LTS - X Stage Module.vi"("Set/Get"=Set_Get_Controls."Set", "Error In"=w480, "Action"=w479, "Cluster In"=w476) -> ("Error Out"=w481:errorcluster)  [unwired: 6 in, 1 out]
                            }
                          }
                        }
                        frame Enabled {
                        }
                      }
                    }
                    frame 1 {
                      # "Y Stage"
                      n145 = disable-structure shown="Enabled" {
                        disable-tunnel: [w491 _] -> w485
                        disable-tunnel: w484 -> [w490 _]
                        disable-tunnel: w483 -> [w489 _]
                        disable-tunnel: w482 -> [w486 _]
                        frame Disabled {
                          n146 = Unbundle By Name(w486) -> ("Y Stage.Model"=w488:T5, "Y Stage.Device SN"=w487:string)
                          n147 = case shown="\"Thorlabs LTS\"" w488 {
                            tunnel: [w492 w499] -> w491
                            tunnel: w490 -> [w492 w498]
                            tunnel: w489 -> [_ w497]
                            tunnel: w487 -> [_ w495]
                            frame "None", Default {
                            }
                            frame "Thorlabs LTS" {
                              n148 = Bundle By Name(cluster=T4 {"Position"=0.0, "Is.Enabled?"=TRUE, "Is.Connected?"=FALSE, "Device SN"="45876539", "AccelerationMaximum"=0.0, "VelocityMaximum"=0.0, "Acceleration"=0.0, "Velocity"=0.0, "waitTimeout (ms)"=0, "Model"=enum."Thorlabs LTS", "Is.Homed?"=FALSE, "MOVE"=FALSE} ("Cluster In"), "Device SN"=w495) -> (w494:T4)
                              n149 = call "Thorlabs LTS - Y Stage Module.vi"("Set/Get"=Set_Get_Controls."Set", "Error In"=w498, "Action"=w497, "Cluster In"=w494) -> ("Error Out"=w499:errorcluster)  [unwired: 6 in, 1 out]
                            }
                          }
                        }
                        frame Enabled {
                        }
                      }
                    }
                    frame 2 {
                      # "Z Stage"
                      n150 = disable-structure shown="Enabled" {
                        disable-tunnel: [w509 _] -> w503
                        disable-tunnel: w502 -> [w508 _]
                        disable-tunnel: w501 -> [w507 _]
                        disable-tunnel: w500 -> [w504 _]
                        frame Disabled {
                          n151 = Unbundle By Name(w504) -> ("Z Stage.Model"=w506:T5, "Z Stage.Device SN"=w505:string)
                          n152 = case shown="\"Thorlabs MLJ\"" w506 {
                            tunnel: [w510 w517] -> w509
                            tunnel: w508 -> [w510 w516]
                            tunnel: w507 -> [_ w515]
                            tunnel: w505 -> [_ w513]
                            frame "None", Default {
                            }
                            frame "Thorlabs MLJ" {
                              n153 = Bundle By Name(cluster=T4 {"Position"=0.0, "Is.Enabled?"=TRUE, "Is.Connected?"=FALSE, "Device SN"="45876539", "AccelerationMaximum"=0.0, "VelocityMaximum"=0.0, "Acceleration"=0.0, "Velocity"=0.0, "waitTimeout (ms)"=0, "Model"=enum."Thorlabs MLJ", "Is.Homed?"=FALSE, "MOVE"=FALSE} ("Cluster In"), "Device SN"=w513) -> (w512:T4)
                              n154 = call "Thorlabs MLJ - Z Stage Module.vi"("Set/Get"=Set_Get_Controls."Set", "Error In"=w516, "Action"=w515, "Cluster In"=w512) -> ("Error Out"=w517:errorcluster)  [unwired: 6 in, 1 out]
                            }
                          }
                        }
                        frame Enabled {
                        }
                      }
                    }
                    frame 3 {
                      # "Vibratome Motor"
                      n155 = call "MCDC3006 Module.vi"("Actions"=T12."Close Session", "Error In"=w518) -> ("Error Out"=w520:errorcluster)  [unwired: 5 in, 4 out]
                      n156 = call <vilib>:"Clear Errors.vi"("error in (no error)"=w520) -> ("error out"=w519:errorcluster)  [unwired: 5 in, 1 out]
                    }
                  }
                }
                n157 = Merge Errors(w457) -> (w455:errorcluster)
              }
              frame Disabled {
                w522 = Set_Get_Controls."Set" ("Set/Get")
                w526 = Motion_Translation_Module_Control."Uninit" ("Action")
                n158 = call "XYZ Table Stage Module.vi"("Set/Get"=w522, "Action"=w526, "Error In"=w534, "Axis"=enum16{"X Axis", "Y Axis", "Z Axis"}."X Axis") -> ("Error Out"=w533:errorcluster)  [unwired: 6 in, 1 out]
                n159 = call "XYZ Table Stage Module.vi"("Set/Get"=w522, "Action"=w526, "Error In"=w533, "Axis"=enum16{"X Axis", "Y Axis", "Z Axis"}."Y Axis") -> ("Error Out"=w532:errorcluster)  [unwired: 6 in, 1 out]
                n160 = call "XYZ Table Stage Module.vi"("Set/Get"=w522, "Action"=w526, "Error In"=w532, "Axis"=enum16{"X Axis", "Y Axis", "Z Axis"}."Z Axis") -> ("Error Out"=w529:errorcluster)  [unwired: 6 in, 1 out]
                n161 = call "MCDC3006 Module.vi"("Actions"=T12."Disable Motor", "Error In"=w529) -> ("Error Out"=w528:errorcluster)  [unwired: 5 in, 4 out]
                n162 = call "MCDC3006 Module.vi"("Actions"=T12."Close Session", "Error In"=w528) -> ("Error Out"=w527:errorcluster)  [unwired: 5 in, 4 out]
              }
            }
          }
          frame "Finished" {
            n163 = call "Inline Wait.vi"("Error In"=w538, "milliseconds to wait"=u32 1000) -> ("Error Out"=w537:errorcluster)  [unwired: 9 in]
          }
        }
        n164 = case shown="No Error" w22 {
          selector: w22 -> [w28 w29]
          tunnel: [w28 w29] -> w21
          tunnel: w20 -> [w27 w32]
          tunnel: [w26 w30] -> w19
          frame No Error {
            n165 = Delete From Array(array=w27, index=0) -> (array with subset deleted=w26:string[])  [unwired: 1 in, 1 out]
          }
          frame Error {
            n166 = Build Array (concatenate)("Error", w32) -> (w30:string[])
          }
        }
      }
    }
    frame Error {
    }
  }
  "error out" <- w4
